vi "Determine Column Type.vi"(8 "error in (no error)":errorcluster, 11 "Field Factory in":refnum<class "Field Factory.lvclass">) -> (0 "error out":errorcluster, 2 "Column":refnum<class "Composed Column.lvclass">, 3 "Field Factory out":refnum<class "Field Factory.lvclass">)   [LabVIEW 2020, in "Composed Fields.lvlib" / "Field Factory.lvclass"]
uses:
  Field Factory.lvclass
  C:/Users/User/Desktop/Raman Program/Database OOP/source/Database OOP/Column Libraries/Column Configuration/Composed Column Factory.lvclass
  Column/Composed Column.lvclass
  Column Configuration/Composed Column Factory.lvclass/Composed Column Factory.ctl
  FK Field/FK Field.lvclass
  C:/Users/User/Desktop/Raman Program/Database OOP/source/Database OOP/Column Libraries/Composed Field/Composed Field.lvclass
  Composed Field/Composed Field.lvclass
  C:/Users/User/Desktop/Raman Program/Database OOP/source/Database OOP/Column Libraries/Column/Composed Column.lvclass
  Basic Columns/Column Configuration/Basic Column Configuration Class/Column Configuration.lvclass
  Column Configuration/Composed Column Factory.lvclass
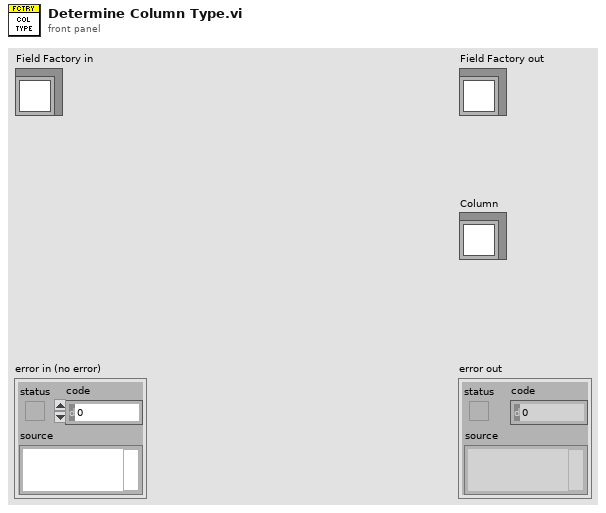
[diagram p1: front panel]
types:
  T1 = typedef "Column Interfaces.lvlib/FK Info.ctl" = cluster{"PK Table":string, "PK Column":string, "PK Display Column":string}
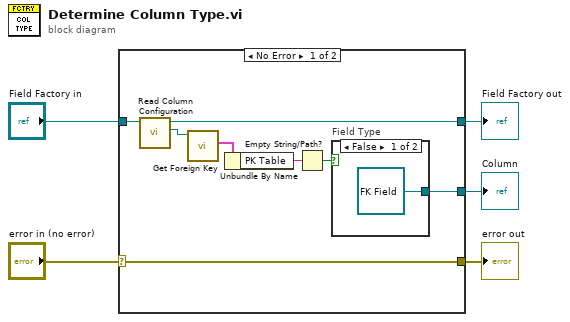
[diagram p0: block diagram]
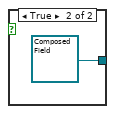
[diagram p2: hidden frame]
diagram:
  n1 = case shown="No Error" "error in (no error)" {
    selector: "error in (no error)" -> [w6 w17]
    tunnel: "Field Factory in" -> [w12 w16]
    tunnel: [w6 w17] -> w3
    tunnel: [w11 w16] -> w2
    tunnel: [w13 _] -> w1
    frame No Error {
      n2 = call "Read Column Configuration.vi"("Composed Column Factory in"=w12) -> ("Column Interfaces.lvlib:Column Configuration.lvclass"=w10:refnum<class "Column Configuration.lvclass">, "Composed Column Factory out"=w11:refnum<class "Field Factory.lvclass">)  [unwired: 8 in, 1 out]
      n3 = call-dynamic "Get Foreign Key.vi"("Basic Column Configuration in"=w10) -> ("FK Info"=w9:T1)  [unwired: 8 in, 2 out]
      n4 = Unbundle By Name(w9) -> ("PK Table"=w8:string)
      n5 = Empty String/Path?(string/path=w8) -> (empty?=w7:bool)
      n6 = case "Field Type" shown="False" w7 {
        tunnel: [refnum<class "FK Field.lvclass"> refnum ("Composed Fields.lvlib:FK Field.lvclass") refnum<class "Composed Field.lvclass"> refnum ("Composed Fields.lvlib:Composed Field.lvclass")] -> w13
        frame False {
        }
        frame True {
        }
      }
    }
    frame Error {
    }
  }
  "error out" <- w3
  "Field Factory out" <- w2
  "Column" <- w1
